vi "set_number_of_pixels.vi"(8 "error in (no error)":errorcluster, 10 "number of pixels":i64, 11 "FPGAWrapperMH120124FrameScan_PXI7813R in":refnum<class "FPGAWrapperMH120124FrameScan_PXI7813R.lvclass">) -> (0 "error out":errorcluster, 3 "FPGAWrapperMH120124FrameScan_PXI7813R out":refnum<class "FPGAWrapperMH120124FrameScan_PXI7813R.lvclass">)   [LabVIEW 2010, in "FPGAWrapperMH120124FrameScan_PXI7813R.lvclass"]
uses:
  FPGAWrapperMH120124FrameScan_PXI7813R.lvclass
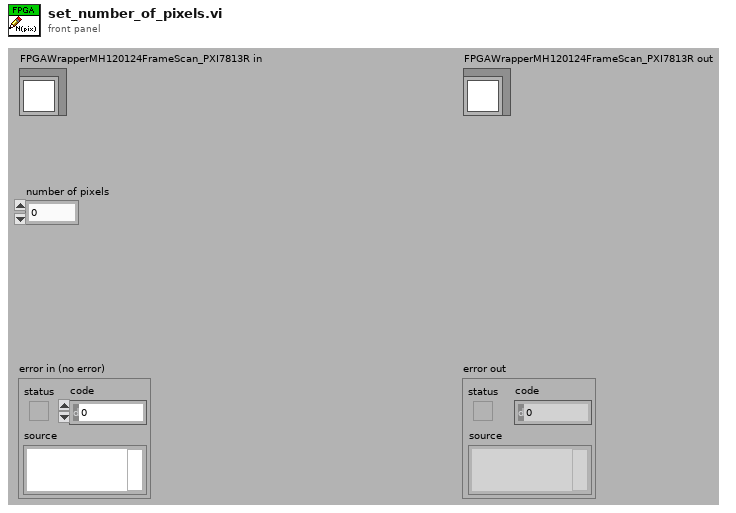
[diagram p1: front panel]
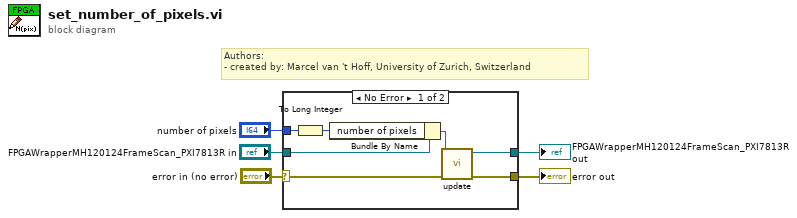
[diagram p0: block diagram]
diagram:
  # "Authors: \n- created by: Marcel van 't Hoff, University of Zurich, Switzerland"
  n1 = case shown="No Error" "error in (no error)" {
    selector: "error in (no error)" -> [w8 w14]
    tunnel: [w7 w14] -> w4
    tunnel: [w9 w13] -> w3
    tunnel: "FPGAWrapperMH120124FrameScan_PXI7813R in" -> [w12 w13]
    tunnel: "number of pixels" -> [w11 _]
    frame No Error {
      n2 = To Long Integer(number=w11) -> (32bit integer=w6:i32)
      n3 = Bundle By Name(cluster=w12, "number of pixels"=w6) -> (w10:refnum<class "FPGAWrapperMH120124FrameScan_PXI7813R.lvclass">)
      n4 = call-dynamic "update.vi"("error in (no error)"=w8, "FPGAWrapperMH120124FrameScan_PXI7813R in"=w10) -> ("error out"=w7:errorcluster, "FPGAWrapperMH120124FrameScan_PXI7813R out"=w9:refnum<class "FPGAWrapperMH120124FrameScan_PXI7813R.lvclass">)  [unwired: 8 in]
    }
    frame Error {
    }
  }
  "error out" <- w4
  "FPGAWrapperMH120124FrameScan_PXI7813R out" <- w3
